vi "MultipleMeasurements_XcpDiffId_Event.vi"() -> ()   [LabVIEW 2019]
doc: "This VI serves as a basic example how to set up a measurement task with several channels.\n\nSelect an A2L data base and a set of measurement channels from it and run the VI. It will display all measurements defined in the chart window. Click Stop when you are done."
uses:
  <vilib>/ECUMC/ECUMC.llb/MC Get Names Type.ctt
  DAQList/DAQList.lvclass/DAQList.ctl
  DAQList/AccessProperties/Read DAQ ref.vi
  A2L_Utility/Private/Find CAN_ID.vi
  DAQList/XnetRead/ProcessMeaSplit.vi
  DAQList/XcpCommand/InitDaqList.vi
  A2L_Utility/Private/ParseNumeric.vi
  DAQList/XnetRead/SubVI_MergeData2.vi
  DAQList/XcpCommand/SendCommands.vi
  DAQList/XcpCommand/FilterCommands.vi
  DAQList/DatabaseGeneration/CreateCluster.vi
  DAQList/DatabaseGeneration/CreateFrames.vi
  DAQList/XnetRead/InitXnet.vi
  DAQList/DatabaseGeneration/CreateSignals_SingleByte.vi
  DAQList/DatabaseGeneration/SubVI_FilterDaqProcessorInfo.vi
  DAQList/DatabaseGeneration/SubVI_FilterDaqResolutionInfo.vi
  DAQList/XnetRead/InitMeaSplitInfo2.vi
  DAQList/DatabaseGeneration/SubVI_ProcessMaxOdtEntrySize.vi
  DAQList/DatabaseGeneration/SubVI_SetMeasProp.vi
  <vilib>/ECUMC/ECUMC.llb/MC Get Property.vi
  <vilib>/ECUMC/ECUMC.llb/MC Get Prop DB File Name.vi
  <vilib>/Utility/file.llb/Read Delimited Spreadsheet.vi
  <vilib>/Utility/file.llb/Read Delimited Spreadsheet (string).vi
  <vilib>/Utility/error.llb/Error Cluster From Error Code.vi
  <vilib>/ECUMC/ECUMC.llb/MC Set Prop Event Channel Name.vi
  <vilib>/xnet/xnet.llb/XNET Create Session.vi
  <vilib>/xnet/xnet.llb/XNET Create Session (Frame Input Stream).vi
  <vilib>/xnet/xnet.llb/XNET Start.vi
  <vilib>/ECUMC/ECUMC.llb/MC DAQ List Initialize.vi
  <vilib>/ECUMC/ECUMC.llb/MC ECU Connect.vi
  <vilib>/ECUMC/ECUMC.llb/MC DAQ Start Stop.vi
  <vilib>/xnet/xnet.llb/XNET Read.vi
  <vilib>/xnet/xnet.llb/XNET Read (Frame CAN).vi
  <vilib>/xnet/xnet.llb/XNET Clear.vi
  <vilib>/ECUMC/ECUMC.llb/MC Get Prop XCP CRO Id.vi
  <vilib>/ECUMC/ECUMC.llb/MC Get Prop XCP DTO Id.vi
  <vilib>/ECUMC/ECUMC.llb/MC Get Prop XCP CAN IO Mode.vi
  <vilib>/ECUMC/ECUMC.llb/MC Get Prop XCP Baud Rate 64.vi
  <vilib>/ECUMC/ECUMC.llb/MC Get Prop XCP FD Baud Rate 64.vi
  <vilib>/xnet/xnet.llb/XNET Database Create Object.vi
  <vilib>/xnet/xnet.llb/XNET Database Create (Cluster).vi
  <vilib>/xnet/xnet.llb/XNET Database Create (Frame).vi
  <vilib>/Utility/file.llb/Application Directory.vi
  <vilib>/xnet/xnet.llb/XNET Database Save.vi
  DAQList/DatabaseGeneration/CreateSignals.vi
  <vilib>/ECUMC/ECUMC.llb/MC Get Prop Meas Address.vi
  <vilib>/xnet/xnet.llb/XNET Database Create (Signal).vi
  <vilib>/xnet/xnet.llb/XNET Database Create (Subframe).vi
  <vilib>/ECUMC/ECUMC.llb/MC Get Prop Meas Data Type.vi
  <vilib>/xnet/xnet.llb/XNET Database Create (Dynamic Signal).vi
  <vilib>/ECUMC/ECUMC.llb/MC Get Prop Meas Comment.vi
  <vilib>/ECUMC/ECUMC.llb/MC Get Prop Meas Scaling Offset.vi
  <vilib>/ECUMC/ECUMC.llb/MC Get Prop Meas Scaling Factor.vi
  <vilib>/ECUMC/ECUMC.llb/MC Get Prop Meas Minimum.vi
  <vilib>/ECUMC/ECUMC.llb/MC Get Prop Meas Maximum.vi
  <vilib>/ECUMC/ECUMC.llb/MC Get Prop Meas Byte Order.vi
  <vilib>/ECUMC/ECUMC.llb/MC Get Prop Meas Unit.vi
  <vilib>/xnet/xnet.llb/XNET Create Session (Signal Input Waveform).vi
  DAQList/TypeDef/Global.vi
  <vilib>/xnet/xnet.llb/XNET Read (Signal Waveform) .vi
  <vilib>/xnet/xnet.llb/XNET Stop.vi
  <vilib>/ECUMC/ECUMC.llb/MC DAQ Clear.vi
  DAQList/DAQList.lvclass
  <vilib>/ECUMC/ECUMC.lvlib
  A2L Utility.lvlib
panel:
  in  "Event Channel":u32(ring) items=["10 ms", "20 ms", "40 ms", "80 ms"]
  in  "Start":bool
  in  "ID Source":bool
  in  "ID Type":bool
  in  "Number of DAQ List":i32=8
  in  "DTO_ID":u32 format="%.0x"
  in  "Measurement List":string[](array[string])=["OneDimTimeSig", "PWM_Signal", "Sinus1", "Sinus2"]
  in  "CAN Interface":refnum<k21>="CAN1"
  in  "Stop":bool
  out "Measurements":waveform(dbl)[](graph)
  in  "A2L Database":path
  # "DISCLAIMER: The attached Code is provided As Is. It has not been tested or validated as a product, for use in a deployed application or system, or for use in hazardous environments. You assume all risks for use of the Code and use of the Code is subject to the Sample Code License Terms which can be found at: http://ni.com/samplecodelicense\n\nImportant Note \n1. This example only works with XCP_ON_CAN.\n2. This example does not work if the DAQ List ID is similar with DTO_ID thus does not work with XCP Demo ECU.\n3. This example does not support dynamic DAQ lists and does not take event channel into consideration."
  # "A2L Database and Connection"
  # "Measurements"
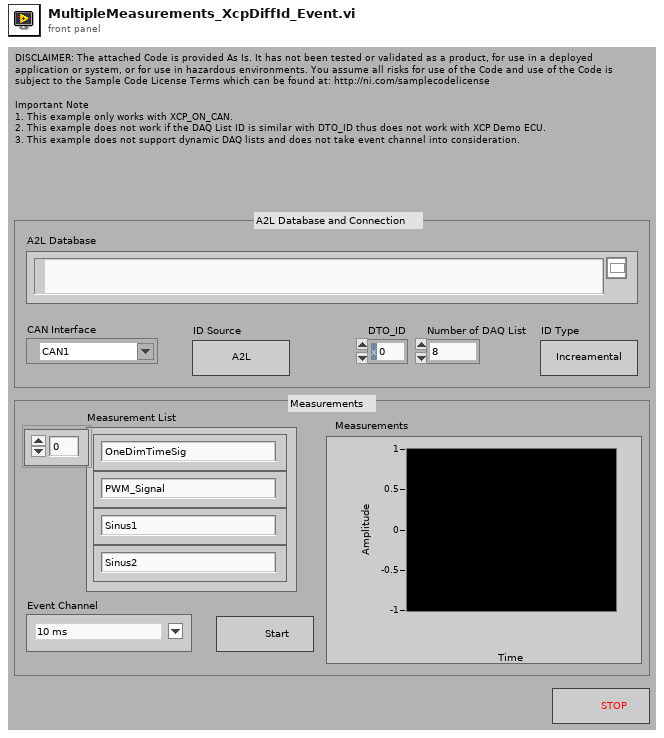
[diagram p1: front panel]
types:
  T1 = typedef "ECUMC.lvlib/MC Get Names Type.ctt" = u32
  T2 = typedef "ECUMC.lvlib/MC Reference.ctt" = u32
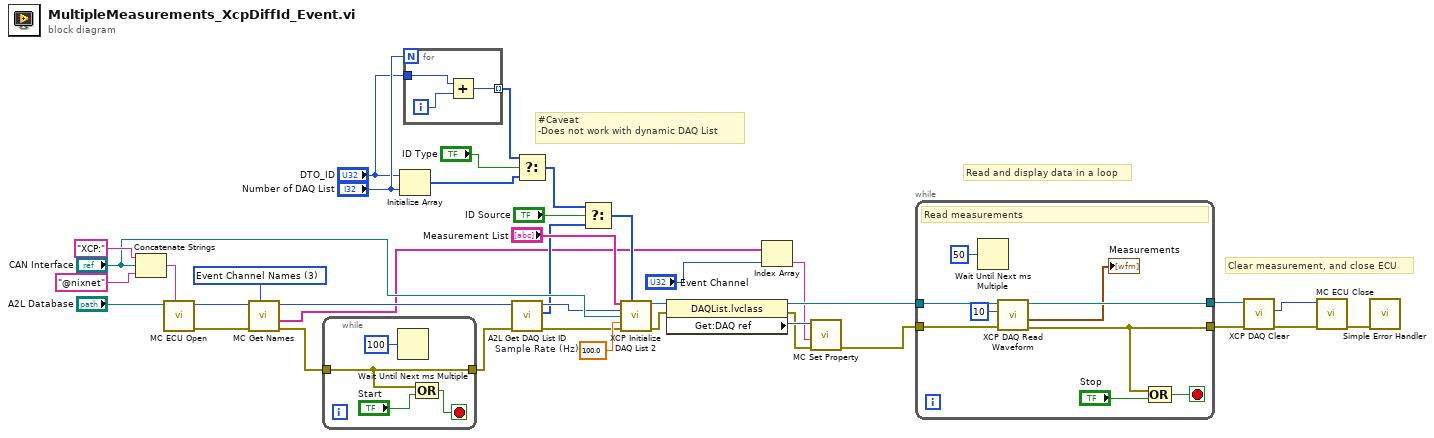
[diagram p0: block diagram]
diagram:
  w8 = T1 3 items=["ECU Names", "Measurement Names", "Characteristic Names", "Event Channel Names", "Defined Pages Names", "Group Names", "Group - Subgroup Names", "Group - Measurement Names", "Group - Characteristic Names", "Function Names", "Function - DefCharacteristic Names", "Function - RefCharacteristic Names", "Function - InMeasurement Names", "Function - OutMeasurement Names", "Function - LocMeasurement Names", "Function - SubFunction Names", "Group - Function List Names", "XCP on CAN - Transport Layer Instance Names", "XCP on TCP - Transport Layer Instance Names", "XCP on UDP - Transport Layer Instance Names"] ("type")
  w22 = 100.0  # Sample Rate (Hz)
  # "Clear measurement, and close ECU"
  # "Read and display data in a loop"
  # "#Caveat\n-Does not work with dynamic DAQ List"
  n1 = Concatenate Strings("XCP:" ("string"), "CAN Interface", "@nixnet" ("string")) -> (w37:string)
  n2 = call <vilib>:"MC ECU Open.vi"("protocol and interface"=w37, "DB path"="A2L Database") -> ("error out"=w1:errorcluster, "ECU ref out"=w5:T2)  [unwired: 1 in, 7 out]
  n3 = call <vilib>:"MC Get Names.vi"("type"=w8, "error in"=w1, "reference in"=w5) -> ("error out"=w6:errorcluster, "names list out"=w3:string[], "reference out"=w4:T2)  [unwired: 1 in, 5 out]
  n4 = while {
    tunnel: w6 -> [w40]
    tunnel: [w40] -> w7
    stop <- w41 stop-if-true
    n5 = Wait Until Next ms Multiple(millisecond multiple=u32 100) -> ()  [unwired: 1 out]
    n6 = Compound Arithmetic op=OR(w40, "Start") -> (w41:bool)
  }
  n7 = Initialize Array("DTO_ID", "Number of DAQ List") -> (w32:u32[])
  n8 = for {
    N: "Number of DAQ List" -> [_]
    tunnel: "DTO_ID" -> [w45]
    tunnel: [w43] -> w29 mode=indexing
    i -> [w44]
    n9 = Add(x=w45, y=w44) -> (x+y=w43:u32)
  }
  n10 = call "A2L Get DAQ List ID.vi"("error in (no error)"=w7, "ECU ref in"=w4) -> ("error out"=w19:errorcluster, "DAQ List IDs"=w16:u32[], "ECU ref out"=w20:T2)  [unwired: 7 in]
  n11 = Select(t=w29, s="ID Type", f=w32) -> (s? t:f=w18:u32[])
  n12 = Select(t=w18, s="ID Source", f=w16) -> (s? t:f=w17:u32[])
  n13 = call "XCP Initialize DAQ List 2.vi"("Measurement List"="Measurement List", "DTO IDs"=w17, "ECU ref in"=w20, "CAN Interface"="CAN Interface", "Sample Rate (10 Hz)"=w22, "error in (no error)"=w19) -> ("DAQList out"=w15:refnum<class "DAQList.lvclass">, "error out"=w14:errorcluster)  [unwired: 8 in]
  n14 = property class="DAQList.lvclass"(reference=w15, error in=w14) -> (reference out=w13:refnum<class "DAQList.lvclass">, error out=w11:errorcluster, "Get:DAQ ref"=w12:T2)
  n15 = Index Array(array=w3, index="Event Channel") -> (element=w2:string)
  n16 = call-poly <vilib>:"MC Set Property.vi"("error in"=w11, "event channel name"=w2, "reference in"=w12) -> ("error out"=w10:errorcluster)  [unwired: 1 in, 7 out]
  n17 = while {
    tunnel: [w49] -> w24
    tunnel: w13 -> [w48]
    tunnel: w10 -> [w51]
    tunnel: [w50] -> w27
    stop <- w54 stop-if-true
    # "Read measurements"
    n18 = Wait Until Next ms Multiple(millisecond multiple=u32 50) -> ()  [unwired: 1 out]
    n19 = call "XCP DAQ Read Waveform.vi"("error in (no error)"=w51, "Number of Sample"=10, "DAQList in"=w48) -> ("error out"=w50:errorcluster, "Data"=→"Measurements":waveform(dbl)[], "DAQList out"=w49:refnum<class "DAQList.lvclass">)  [unwired: 5 in, 1 out]
    n20 = Compound Arithmetic op=OR(w50, "Stop") -> (w54:bool)
  }
  n21 = call "XCP DAQ Clear.vi"("error in (no error)"=w27, "DAQList in"=w24) -> ("error out"=w26:errorcluster, "ECU ref out"=w25:T2)  [unwired: 8 in]
  n22 = call <vilib>:"MC ECU Close.vi"("error in"=w26, "ECU ref in"=w25) -> ("error out"=w34:errorcluster)  [unwired: 9 out]
  n23 = call <vilib>:"Simple Error Handler.vi"("error in (no error)"=w34) -> ()  [unwired: 1 in, 8 out]
